vi "proyecto.vi"() -> ()   [LabVIEW 2012]
uses:
  <vilib>/Analysis/2dsp.llb/Real FFT.vi
  <vilib>/Analysis/NI_AALPro.lvlib
  <vilib>/measure/NI_MABase.lvlib
panel:
  in  "spectral amplitude":dbl=1.0 format="%0.2f"
  in  "Enum 2":T1(ring)
  in  "Enum":T1(ring)
  in  "Boolean":bool
  out "Transformada Sumada":dbl[](graph)
  out "Señal Sumada":dynamicdata(graph)
  out "Transformada Dos":dbl[](graph)
  out "Señal Dos":dynamicdata(graph)
  in  "Amplitud 2":dbl
  in  "Frecuencia 2":dbl
  out "Transformada Uno":dbl[](graph)
  out "Señal Uno":dynamicdata(graph)
  in  "Amplitud":dbl
  in  "Frecuencia":dbl
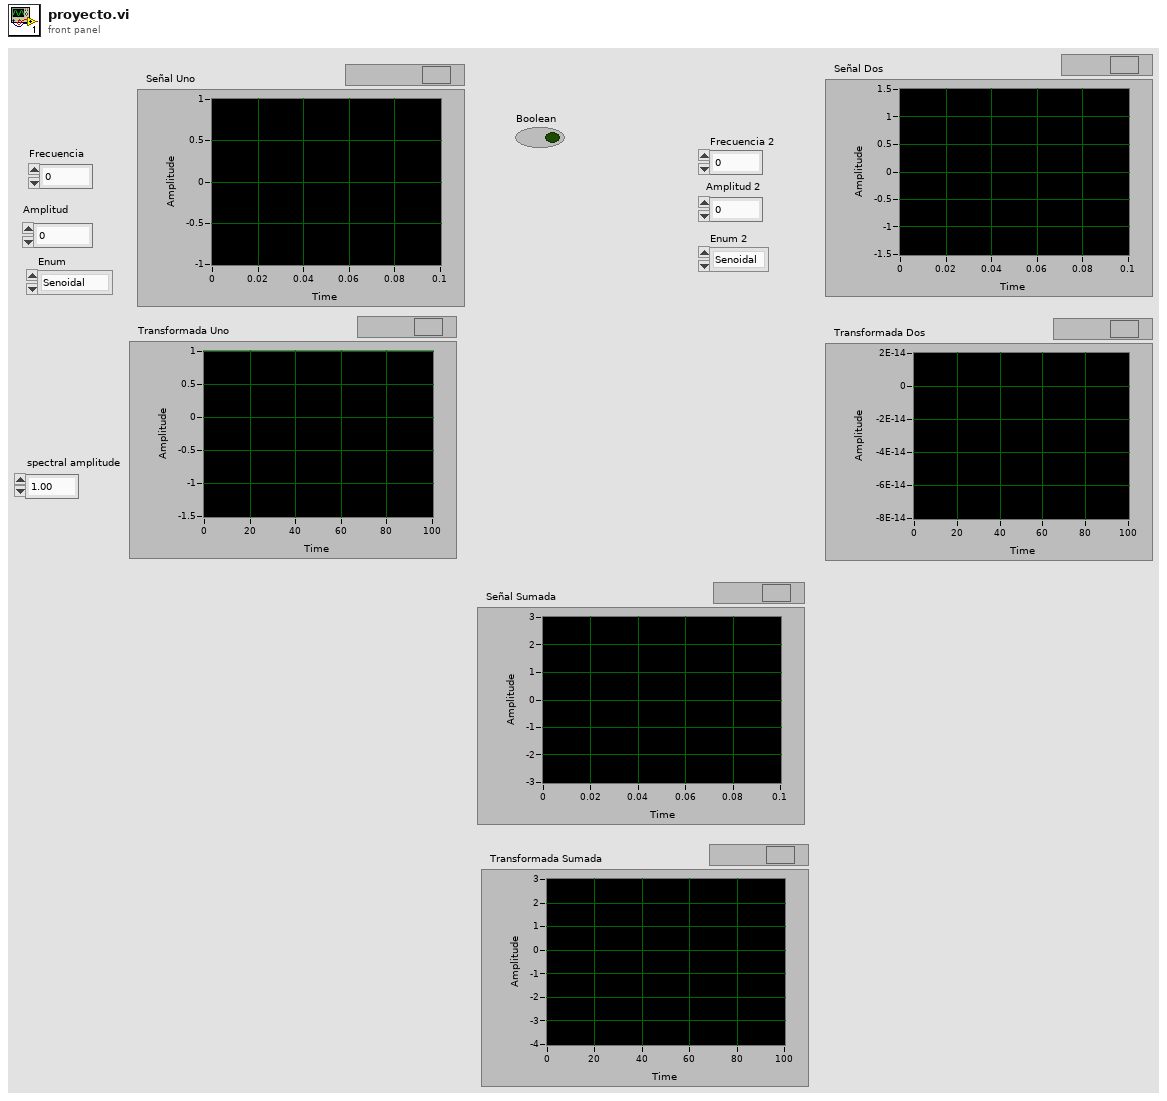
[diagram p1: front panel]
types:
  T1 = enum16{"Senoidal", "Cuadrada", "Triangular", "Diente Sierra"}
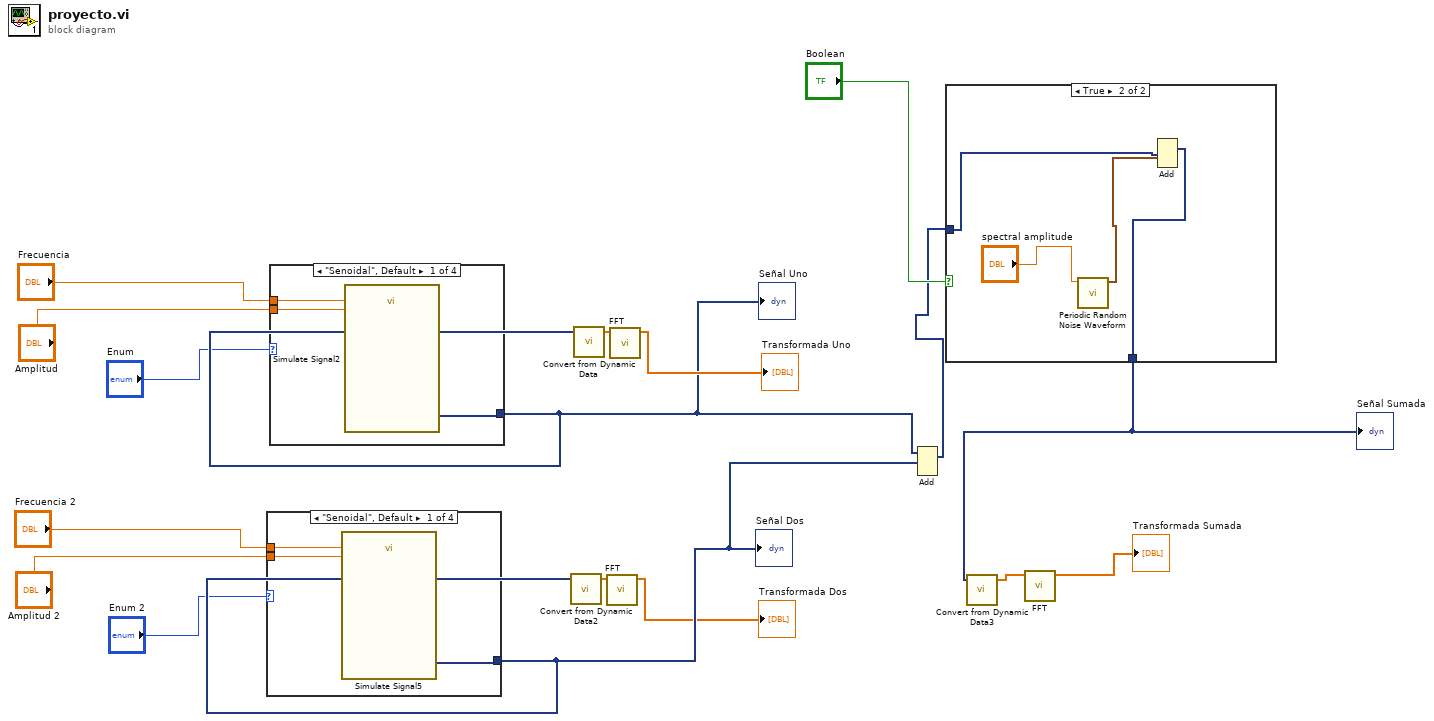
[diagram p0: block diagram]
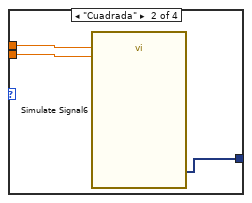
[diagram p3: hidden frame]
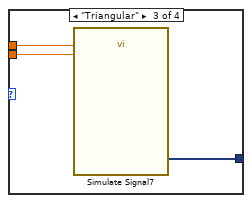
[diagram p4: hidden frame]
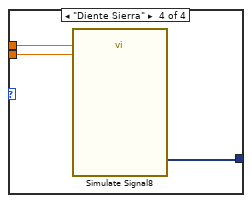
[diagram p5: hidden frame]
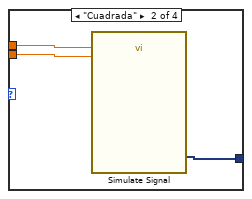
[diagram p6: hidden frame]
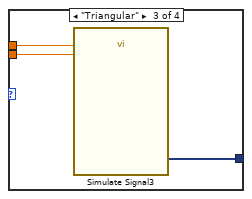
[diagram p7: hidden frame]
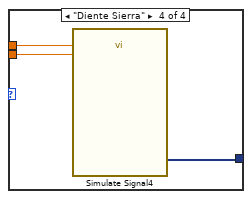
[diagram p8: hidden frame]
diagram:
  n1 = case shown="\"Senoidal\", Default" "Enum 2" {
    tunnel: "Frecuencia 2" -> [w20 w23 w26 w29]
    tunnel: "Amplitud 2" -> [w19 w22 w25 w28]
    tunnel: [w18 w21 w24 w27] -> w10
    frame "Senoidal", Default {
      n2 = call "Simulate Signal5"("Frequency"=w20, "Amplitude"=w19) -> ("Sine"=w18:dynamicdata)  [unwired: 12 in, 1 out]
    }
    frame "Cuadrada" {
      n3 = call "Simulate Signal6"("Frequency"=w23, "Amplitude"=w22) -> ("Square"=w21:dynamicdata)  [unwired: 12 in, 1 out]
    }
    frame "Triangular" {
      n4 = call "Simulate Signal7"("Frequency"=w26, "Amplitude"=w25) -> ("Triangle"=w24:dynamicdata)  [unwired: 12 in, 1 out]
    }
    frame "Diente Sierra" {
      n5 = call "Simulate Signal8"("Frequency"=w29, "Amplitude"=w28) -> ("Sawtooth"=w27:dynamicdata)  [unwired: 12 in, 1 out]
    }
  }
  "Señal Dos" <- w10
  n6 = case shown="\"Senoidal\", Default" "Enum" {
    tunnel: "Frecuencia" -> [w32 w35 w38 w41]
    tunnel: "Amplitud" -> [w31 w34 w37 w40]
    tunnel: [w30 w33 w36 w39] -> w9
    frame "Senoidal", Default {
      n7 = call "Simulate Signal2"("Frequency"=w32, "Amplitude"=w31) -> ("Sine"=w30:dynamicdata)  [unwired: 12 in, 1 out]
    }
    frame "Cuadrada" {
      n8 = call "Simulate Signal"("Frequency"=w35, "Amplitude"=w34) -> ("Square"=w33:dynamicdata)  [unwired: 12 in, 1 out]
    }
    frame "Triangular" {
      n9 = call "Simulate Signal3"("Frequency"=w38, "Amplitude"=w37) -> ("Triangle"=w36:dynamicdata)  [unwired: 12 in, 1 out]
    }
    frame "Diente Sierra" {
      n10 = call "Simulate Signal4"("Frequency"=w41, "Amplitude"=w40) -> ("Sawtooth"=w39:dynamicdata)  [unwired: 12 in, 1 out]
    }
  }
  "Señal Uno" <- w9
  n11 = call "Convert from Dynamic Data2"("Dynamic Data Type"=w10) -> ("Array"=w11:dbl[])  [unwired: 3 in]
  n12 = call "Convert from Dynamic Data"("Dynamic Data Type"=w9) -> ("Array"=w14:dbl[])  [unwired: 3 in]
  n13 = call-poly <vilib>:"FFT.vi"("X"=w11) -> ("FFT {X}"=→"Transformada Dos":cdb[])  [unwired: 9 in, 1 out]
  n14 = call-poly <vilib>:"FFT.vi"("X"=w14) -> ("FFT {X}"=→"Transformada Uno":cdb[])  [unwired: 9 in, 1 out]
  n15 = Add(1:w10, 2:w9) -> (0:w3:dynamicdata)  [unwired: 1 in, 1 out]
  n16 = case shown="True" "Boolean" {
    tunnel: w3 -> [w42 w46]
    tunnel: [w42 w43] -> w1
    frame False {
    }
    frame True {
      n17 = call <vilib>:"Periodic Random Noise Waveform.vi"("spectral amplitude"="spectral amplitude") -> ("signal out"=w44:waveform(dbl))  [unwired: 9 in, 1 out]
      n18 = Add(1:w46, 2:w44) -> (0:w43:dynamicdata)  [unwired: 1 in, 1 out]
    }
  }
  "Señal Sumada" <- w1
  n19 = call "Convert from Dynamic Data3"("Dynamic Data Type"=w1) -> ("Array"=w2:dbl[])  [unwired: 3 in]
  n20 = call-poly <vilib>:"FFT.vi"("X"=w2) -> ("FFT {X}"=→"Transformada Sumada":cdb[])  [unwired: 9 in, 1 out]
